vi "HDF5_clust2group.vi"(7 "group name":string="settings", 8 "error in":errorcluster, 9 "cluster in":variant, 11 "ref in":T1 format="%.0x") -> (0 "error out":errorcluster, 3 "ref out":T1 format="%.0x")   [LabVIEW 2015]
uses:
  <vilib>/addons/h5labview2/base/hid_t.ctl
  <vilib>/addons/h5labview2/dataset/H5D.lvlib
  <vilib>/addons/h5labview2/group/H5G.lvlib
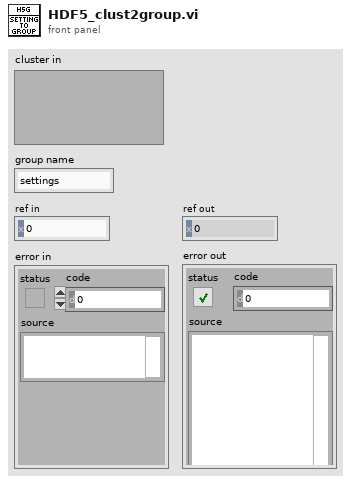
[diagram p1: front panel]
types:
  T1 = typedef "hid_t.ctl" = i32
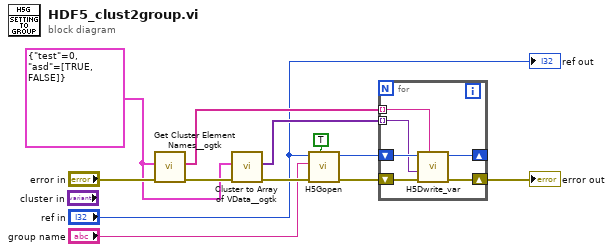
[diagram p0: block diagram]
diagram:
  w1 = cluster{"test":i32, "asd":bool[]} {"test"=0, "asd"=[TRUE, FALSE]}
  n1 = call <userlib>:"Get Cluster Element Names__ogtk.vi"("error in (no error)"="error in", "Cluster"=w1) -> ("error out"=w10:errorcluster, "Element Names"=w7:string[])  [unwired: 8 in]
  n2 = call <userlib>:"Cluster to Array of VData__ogtk.vi"("error in (no error)"=w10, "Cluster"=w1) -> ("error out"=w11:errorcluster, "Array of VData"=w8:variant[])  [unwired: 8 in]
  n3 = call <vilib>:"H5Gopen.vi"("create? (F)"=TRUE, "error in (no error)"=w11, "name"="group name", "ref in"="ref in") -> ("error out"=w12:errorcluster, "group out"=w6:T1)  [unwired: 6 in]
  n4 = for {
    shift-right: [w15] -> _
    shift-left: w6 -> [w18]
    shift-right: [w16] -> w2
    shift-left: w12 -> [w17]
    tunnel: w8 -> [w13] mode=indexing
    tunnel: w7 -> [w14] mode=indexing
    n5 = call <vilib>:"H5Dwrite_var.vi"("dataset name"=w14, "error in (no error)"=w17, "data"=w13, "ref in"=w18) -> ("error out"=w16:errorcluster, "ref out"=w15:T1)  [unwired: 5 in, 1 out]
  }
  "error out" <- w2
  "ref out" <- "ref in"
